vi "数据和索引.vi"(11 "data out":string) -> (0 "颜色":u32, 1 "显示数据":string, 2 "编号":i32, 4 "NG?":bool, 5 "条码":string)   [LabVIEW 2014]
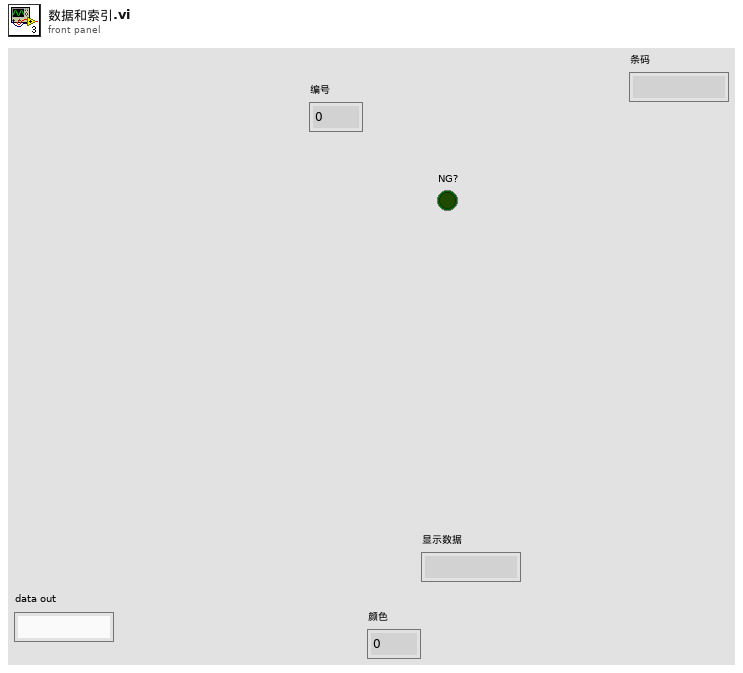
[diagram p1: front panel]
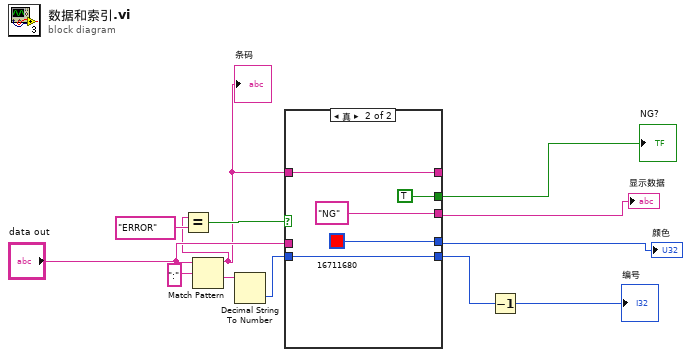
[diagram p0: block diagram]
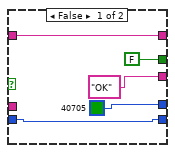
[diagram p2: hidden frame]
diagram:
  n1 = Match Pattern(string="data out", regular expression=":" ("正则表达式")) -> (before substring=w3:string, after substring=w12:string)  [unwired: 1 in, 2 out]
  "条码" <- w3
  n2 = Equal?(x=w3, y="ERROR") -> (x = y?=w10:bool)
  n3 = Decimal String To Number(string=w12) -> (number=w11:i32)  [unwired: 2 in, 1 out]
  n4 = case shown="真" w10 {
    tunnel: ["OK" "NG"] -> w6
    tunnel: w11 -> [w16 w19]
    tunnel: [w16 w19] -> w2
    tunnel: [u32 40705 u32 16711680] -> w7
    tunnel: "data out" -> [_ _]
    tunnel: [FALSE TRUE] -> w4
    tunnel: w3 -> [w13 w18]
    tunnel: [w13 w18] -> _
    frame False {
    }
    frame True {
    }
  }
  "显示数据" <- w6
  "颜色" <- w7
  "NG?" <- w4
  n5 = Decrement(x=w2) -> (x-1=→"编号":i32)
